vi "testTopic.vi"(8 "error in (no error)":errorcluster) -> (0 "error out":errorcluster)   [LabVIEW 2018]
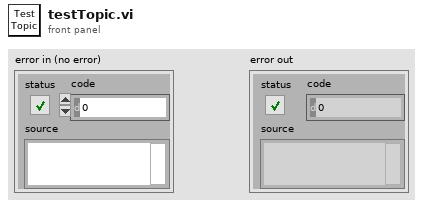
[diagram p1: front panel]
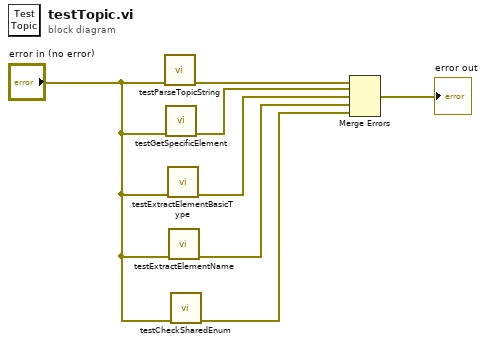
[diagram p0: block diagram]
diagram:
  n1 = call "testParseTopicString.vi"("error in (no error)"="error in (no error)") -> ("error out"=w7:errorcluster)  [unwired: 10 in]
  n2 = call "testGetSpecificElement.vi"("error in (no error)"="error in (no error)") -> ("error out"=w6:errorcluster)  [unwired: 10 in]
  n3 = call "testExtractElementBasicType.vi"("error in (no error)"="error in (no error)") -> ("error out"=w4:errorcluster)  [unwired: 10 in]
  n4 = call "testExtractElementName.vi"("error in (no error)"="error in (no error)") -> ("error out"=w3:errorcluster)  [unwired: 10 in]
  n5 = call "testCheckSharedEnum.vi"("error in (no error)"="error in (no error)") -> ("error out"=w1:errorcluster)  [unwired: 10 in]
  n6 = Merge Errors(w7, w6, w4, w3, w1) -> (→"error out":errorcluster)
